vi "signalchanneltest.vi"() -> ()   [LabVIEW 2021]
uses:
  <userlib>/Nanonis Prog Interface V5/Nanonis Prog Interface.lvlib
panel:
  in  "Signals indexes (0-127)":i8[](array[numeric]) min=0
  out "Value":dbl
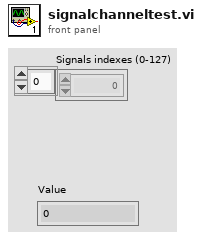
[diagram p1: front panel]
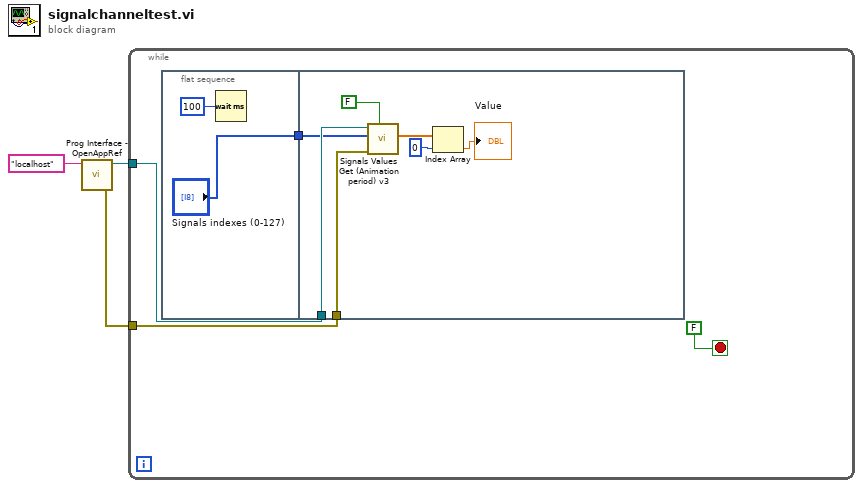
[diagram p0: block diagram]
diagram:
  n1 = call <userlib>:"Prog Interface - OpenAppRef.vi"("Machine name (local machine IP)"="localhost" ("machine name (localhost)")) -> ("Error out"=w1:errorcluster, "Application reference"=w2:refnum<vi>)  [unwired: 5 in]
  n2 = while {
    tunnel: w2 -> [w6]
    tunnel: w1 -> [w5]
    stop <- FALSE stop-if-true
    n3 = flat-sequence {
      tunnel: ["Signals indexes (0-127)"] -> w4
      tunnel: w6 -> [w13]
      tunnel: w5 -> [w12]
      tunnel: w4 -> [w10]
      frame #0 {
        n4 = Wait (ms)(milliseconds to wait=u32 100) -> ()  [unwired: 1 out]
      }
      frame #1 {
        n5 = call <userlib>:"Signals Values Get (Animation period) v3.vi"("Wait for newest data (F=False)"=FALSE, "error in (no error)"=w12, "Signals indexes (0-127)"=w10, "Application ref in"=w13) -> ("Signals Values"=w16:sgl[])  [unwired: 4 in, 2 out]
        n6 = Index Array(array=w16, index=0) -> (element=→"Value":sgl)
      }
    }
  }
